vi "Point.vi"() -> ()   [LabVIEW 2015]
panel:
  out "Waveform Graph 2":dbl[](graph)
  out "Max Voltage":dbl
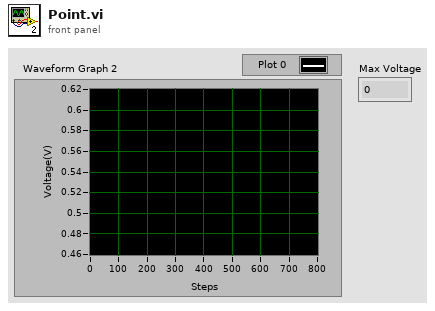
[diagram p1: front panel]
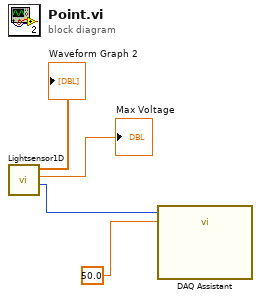
[diagram p0: block diagram]
diagram:
  n1 = call "Lightsensor1D.vi"() -> ("max index(es)"=w3:i32, "max value"=→"Max Voltage":dbl, "Waveform Graph 2"=→"Waveform Graph 2":dbl[])  [unwired: 9 in]
  n2 = call "DAQ Assistant"("number of samples"=w3, "timeout (s)"=50.0) -> ()  [unwired: 16 in, 2 out]
